vi "ShowData.vi"() -> ()   [LabVIEW 2022 SP3]
uses:
  <vilib>/sound2/lvsound2.llb/Sound Data Format.ctl
  <vilib>/sound2/lvsound2.llb/Sampling Mode.ctl
  <vilib>/sound2/lvsound2.llb/Sound Output Write (DBL Single).vi
panel:
  in  "Previous":bool
  in  "Next":bool
  out "Seek":bool
  out "TotSmpls":i64
  in  "PrevBtn":bool
  in  "SkipBtn":bool
  in  "FilePos":i32=8000
  in  "Skip":i32=220000 format="%#_4p"
  out "dt":dbl
  out "PlayBuffer":dbl[](array[numeric])
  out "Cnt":i32
  out "Chunks":i32
  in  "Export":path=path "D:/Temp"
  out "task ID":u32
  out "n":u16=1
  in  "ch":u16
  in  "ch_mask":u16=8000 format="%05b"
  in  "Reload":bool
  in  "SaveWav":bool
  in  "fs":u16=8000
  in  "Play":bool
  in  "Path":path
  out "min":u16
  out "max":u16
  out "Graph":u16[][](graph)
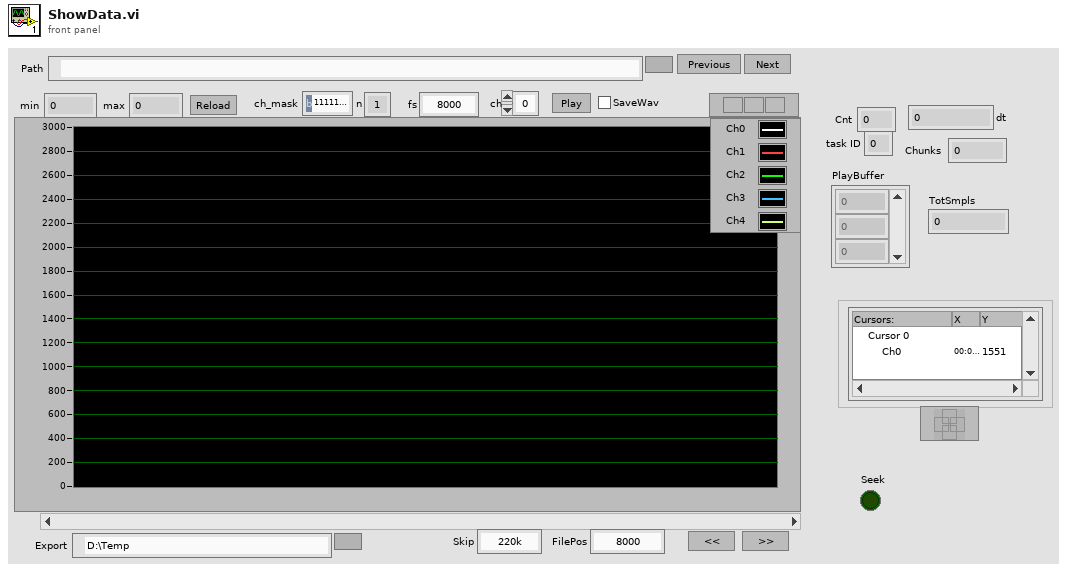
[diagram p1: front panel]
types:
  T1 = enum16{"big-endian, network order", "native, host order", "little-endian"}
  T2 = typedef "Sound Data Format.ctl" = cluster{"sample rate (S/s)":dbl, "number of channels":i32, "bits per sample":i32}
  T3 = typedef "Sampling Mode.ctl" = i32
  T4 = typedef "Sound Output Task ID.ctl" = u32
  T5 = typedef "LVPoint32TypeDef.ctl" = cluster{"Horizontal":i32, "Vertical":i32}
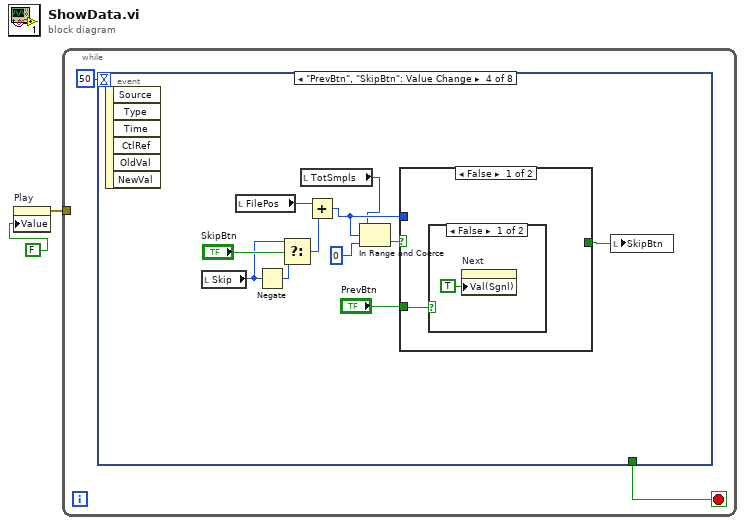
[diagram p0: block diagram]
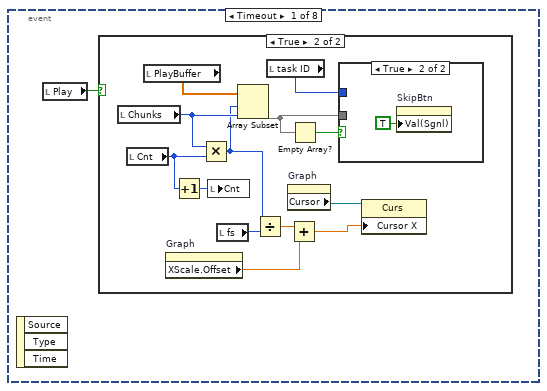
[diagram p2: hidden frame]
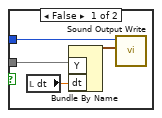
[diagram p4: hidden frame]
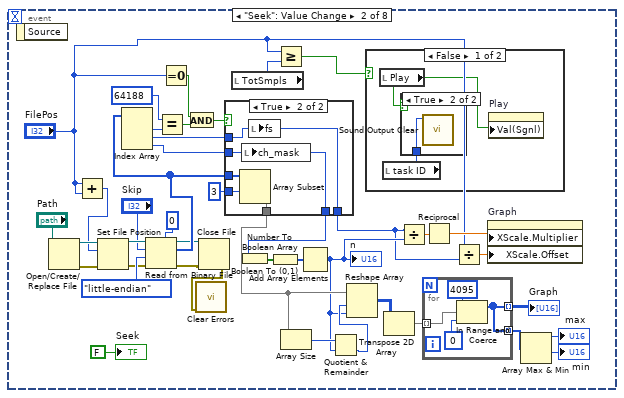
[diagram p5: hidden frame]
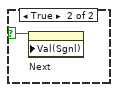
[diagram p7: hidden frame]
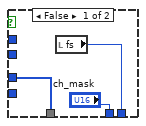
[diagram p8: hidden frame]
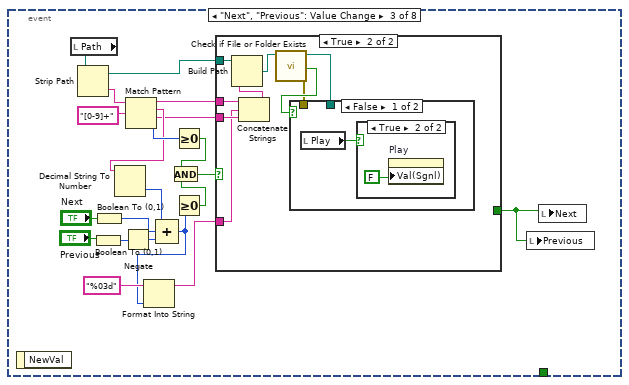
[diagram p9: hidden frame]
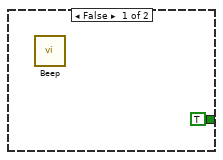
[diagram p10: hidden frame]
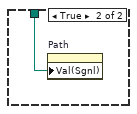
[diagram p12: hidden frame]
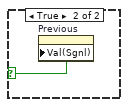
[diagram p13: hidden frame]
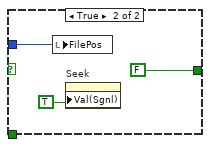
[diagram p14: hidden frame]
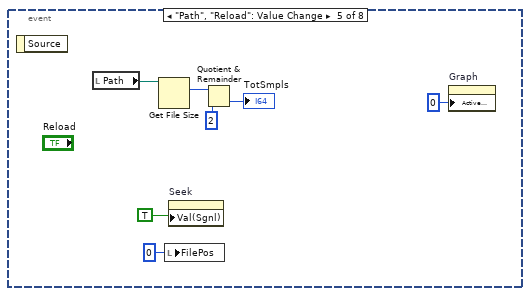
[diagram p15: hidden frame]
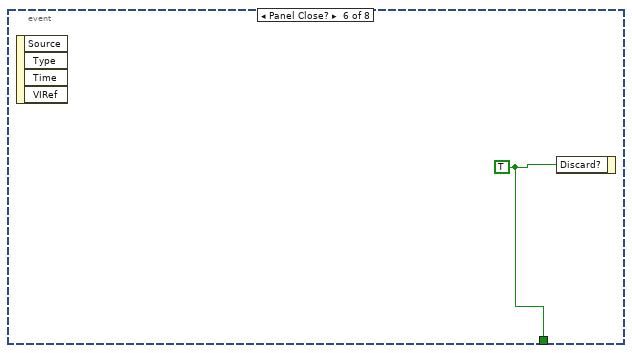
[diagram p16: hidden frame]
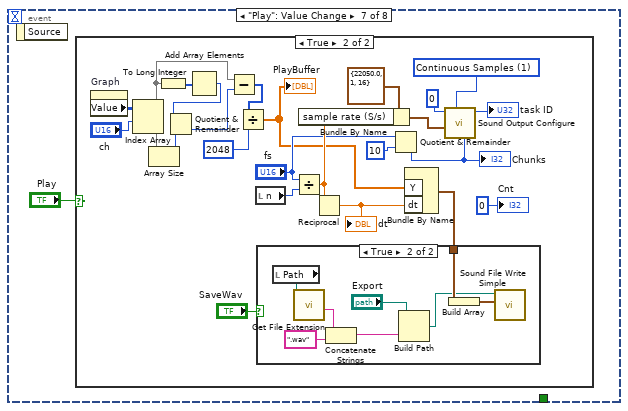
[diagram p17: hidden frame]
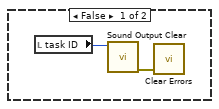
[diagram p18: hidden frame]
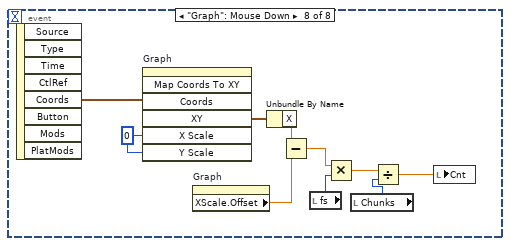
[diagram p20: hidden frame]
diagram:
  n1 = property on="Play" class="Bool (strict)"("Value"=FALSE) -> (error out=w2:errorcluster)  [unwired: 2 in, 1 out]
  n2 = while {
    tunnel: w2 -> [_]
    stop <- w4 stop-if-true
    n3 = event shown="[3] \"PrevBtn\", \"SkipBtn\": Value Change" {
      selector: _ -> [_ _ _ _ _ _ _ _]
      dyn-events: _ -> [_ _ _ _ _ _ _ _]
      timeout: 50 -> [_ _ _ _ _ _ _ _]
      tunnel: [_ _ _ _ _ w140 _ _] -> w4
      event Timeout {
        n4 = event-data() -> ()  [unwired: 1 in, 3 out]
        n5 = local read "Play"() -> (w5:bool)
        n6 = case shown="True" w5 {
          frame False {
          }
          frame True {
            n7 = local read "Chunks"() -> (w17:i32)
            n8 = local read "Cnt"() -> (w13:i32)
            n9 = local read "PlayBuffer"() -> (w18:dbl[])
            n10 = property on="Graph" class="WFGraph (strict)"() -> ("XScale.Offset"=w6:dbl)  [unwired: 2 in, 2 out]
            n11 = Increment(x=w13) -> (x+1=w12:i32)
            n12 = Multiply(x=w17, y=w13) -> (x*y=w10:i32)
            n13 = local write "Cnt"(w12) -> ()
            n14 = local read "fs"() -> (w11:u16)
            n15 = Array Subset(array=w18, index=w10, length=w17) -> (w15:dbl[])
            n16 = Divide(x=w10, y=w11) -> (x/y=w8:dbl)
            n17 = local read "task ID"() -> (w16:u32)
            n18 = property on="Graph" class="WFGraph (strict)"() -> ("Cursor"=w9:refnum<vi>)  [unwired: 2 in, 2 out]
            n19 = Add(x=w8, y=w6) -> (x+y=w7:dbl)
            n20 = Empty Array?(array=w15) -> (empty?=w14:bool)
            n21 = case shown="True" w14 {
              tunnel: w16 -> [w20 _]
              tunnel: w15 -> [w19 _]
              frame False {
                n22 = local read "dt"() -> (w22:dbl)
                n23 = Bundle By Name("Y"=w19, "dt"=w22) -> (w21:waveform(dbl))  [unwired: 1 in]
                n24 = call-poly <vilib>:"Sound Output Write.vi"("data"=w21, "task ID"=w20) -> ()  [unwired: 8 in, 2 out]
              }
              frame True {
                n25 = property on="SkipBtn" class="Bool (strict)"("Val(Sgnl)"=TRUE) -> ()  [unwired: 2 in, 2 out]
              }
            }
            n26 = property class="Curs"(reference=w9, "Cursor X"=w7) -> ()  [unwired: 1 in, 2 out]
          }
        }
      }
      event "Seek": Value Change {
        n27 = event-data() -> ()  [unwired: 1 in, 1 out]
        n28 = Open/Create/Replace File(file path (use dialog)="Path") -> (refnum out=w45:refnum<file>, error out=w42:errorcluster)  [unwired: 5 in, 1 out]
        n29 = Add(x="FilePos", y="FilePos") -> (x+y=w44:i32)
        n30 = Set File Position(offset (in bytes) (0)=w44, refnum=w45, error in=w42) -> (refnum out=w43:refnum<file>, error out=w27:errorcluster)  [unwired: 1 in]
        n31 = Read from Binary File(5:u16 0, 8:w27, 9:T1."little-endian" ("byte order (0:big-endian, network order)"), 10:"Skip", 11:w43) -> (0:w36:errorcluster, 2:w46:u16[], 3:w37:refnum<file>)  [unwired: 1 in, 1 out]
        n32 = Index Array(array=w46) -> (element #1=w59:u16, element #2=w57:u16, element #3=w56:u16)  [unwired: 3 in]
        n33 = Equal?(x=u16 64188, y=w59) -> (x = y?=w58:bool)
        n34 = Equal To 0?(x="FilePos") -> (x = 0?=w39:bool)
        n35 = And(x=w39, y=w58) -> (x .and. y?=w41:bool)
        n36 = Close File(refnum=w37, error in=w36) -> (error out=w28:errorcluster)  [unwired: 1 out]
        n37 = call <vilib>:"Clear Errors.vi"("error in (no error)"=w28) -> ()  [unwired: 5 in, 2 out]
        n38 = case shown="True" w41 {
          tunnel: w57 -> [_ w73]
          tunnel: w46 -> [w72 w77]
          tunnel: w56 -> [_ w74]
          tunnel: 3 ("index") -> [_ w76]
          tunnel: [w72 w75] -> w50
          tunnel: ["ch_mask" w74] -> w49
          tunnel: [w70 w73] -> w30
          frame False {
            n39 = local read "fs"() -> (w70:u16)
          }
          frame True {
            n40 = Array Subset(array=w77, index=w76) -> (w75:u16[])  [unwired: 1 in]
            n41 = local write "ch_mask"(w74) -> ()
            n42 = local write "fs"(w73) -> ()
          }
        }
        n43 = local read "TotSmpls"() -> (w35:i64)
        n44 = Number To Boolean Array(number=w49) -> (Boolean array=w54:bool[])
        n45 = Boolean To (0,1)(Boolean=w54) -> (0, 1=w53:i16[])
        n46 = Greater Or Equal?(x="FilePos", y=w35) -> (x >= y?=w25:bool)
        n47 = Array Size(array=w50) -> (size(s)=w52:i32)
        n48 = Add Array Elements(numeric array=w53) -> (sum=w34:i16)
        "n" <- w34
        n49 = Quotient & Remainder(x=w52, y=w34) -> (floor(x/y)=w48:i32)  [unwired: 1 out]
        n50 = Reshape Array(w50, w48, w34) -> (w51:u16[][])
        n51 = case shown="False" w25 {
          selector: w25 -> [_ w69]
          frame False {
            n52 = local read "Play"() -> (w66:bool)
            n53 = local read "task ID"() -> (w67:u32)
            n54 = case shown="True" w66 {
              tunnel: w67 -> [_ w68]
              frame False {
              }
              frame True {
                n55 = call <vilib>:"Sound Output Clear.vi"("task ID"=w68) -> ()  [unwired: 10 in, 1 out]
              }
            }
            n56 = property on="Play" class="Bool (strict)"("Val(Sgnl)"=w66) -> ()  [unwired: 2 in, 2 out]
          }
          frame True {
            n57 = property on="Next" class="Bool (strict)"("Val(Sgnl)"=w69) -> ()  [unwired: 2 in, 2 out]
          }
        }
        n58 = Transpose 2D Array(2D array=w51) -> (transposed array=w61:u16[][])
        n59 = Divide(x=w30, y=w34) -> (x/y=w33:dbl)
        n60 = for {
          tunnel: w61 -> [w79] mode=indexing
          tunnel: [w78] -> w63 mode=indexing
          tunnel: [w78] -> w62 mode=concatenating
          n61 = In Range and Coerce(upper limit=u16 4095 ("x"), x=w79, lower limit=u16 0 ("x")) -> (coerced(x)=w78:u16[])  [unwired: 1 out]
        }
        "Graph" <- w63
        n62 = Reciprocal(x=w33) -> (1/x=w32:dbl)
        n63 = Divide(x="FilePos", y=w30) -> (x/y=w31:dbl)
        n64 = property on="Graph" class="WFGraph (strict)"("XScale.Multiplier"=w32, "XScale.Offset"=w31) -> ()  [unwired: 2 in, 2 out]
        n65 = Array Max & Min(array=w62) -> (max value=→"max":u16, min value=→"min":u16)  [unwired: 2 out]
        "Seek" <- FALSE
      }
      event "Next", "Previous": Value Change {
        n66 = event-data() -> ()  [unwired: 1 in, 1 out]
        n67 = local read "Path"() -> (w97:path)
        n68 = Strip Path(path=w97) -> (stripped path=w91:path, name=w96:string)
        n69 = Boolean To (0,1)(Boolean="Previous") -> (0, 1=w100:i16)
        n70 = Boolean To (0,1)(Boolean="Next") -> (0, 1=w98:i16)
        n71 = Negate(x=w100) -> (-x=w99:i16)
        n72 = Match Pattern(string=w96, regular expression="[0-9]+") -> (before substring=w90:string, match substring=w93:string, after substring=w89:string, offset past match=w94:i32)  [unwired: 1 in]
        n73 = Decimal String To Number(string=w93) -> (number=w92:i32)  [unwired: 2 in, 1 out]
        n74 = Compound Arithmetic op=ADD(w92, w98, w99) -> (w83:i32)
        n75 = Format Into String(format string="%03d", w83) -> (resulting string=w87:string)  [unwired: 2 in, 1 out]
        n76 = Greater Or Equal To 0?(x=w94) -> (x >= 0?=w85:bool)
        n77 = Greater Or Equal To 0?(x=w83) -> (x >= 0?=w84:bool)
        n78 = And(x=w85, y=w84) -> (x .and. y?=w86:bool)
        n79 = case shown="True" w86 {
          tunnel: w91 -> [_ w112]
          tunnel: w90 -> [_ w110]
          tunnel: w89 -> [_ w109]
          tunnel: w87 -> [_ w108]
          tunnel: [TRUE _] -> w82
          frame False {
            n80 = call <vilib>:"Beep.vi"() -> ()  [unwired: 12 in]
          }
          frame True {
            n81 = Concatenate Strings(w110, w108, w109) -> (w111:string)
            n82 = Build Path(base path=w112, name or relative path=w111) -> (appended path=w107:path)
            n83 = call <vilib>:"Check if File or Folder Exists.vi"("path"=w107) -> ("error out"=w105:errorcluster, "file or folder exists?"=w106:bool, "dup path"=w104:path)  [unwired: 8 in]
            n84 = case shown="False" w106 {
              tunnel: w105 -> [_ _]
              tunnel: w104 -> [_ w115]
              frame False {
                n85 = local read "Play"() -> (w113:bool)
                n86 = case shown="True" w113 {
                  frame False {
                  }
                  frame True {
                    n87 = property on="Play" class="Bool (strict)"("Val(Sgnl)"=FALSE) -> ()  [unwired: 2 in, 2 out]
                  }
                }
              }
              frame True {
                n88 = property on="Path" class="Path"("Val(Sgnl)"=w115) -> ()  [unwired: 2 in, 2 out]
              }
            }
          }
        }
        n89 = local write "Previous"(w82) -> ()
        n90 = local write "Next"(w82) -> ()
      }
      event "PrevBtn", "SkipBtn": Value Change {
        n91 = event-data() -> ()  [unwired: 1 in, 6 out]
        n92 = local read "Skip"() -> (w123:i32)
        n93 = local read "FilePos"() -> (w126:i32)
        n94 = Negate(x=w123) -> (-x=w125:i32)
        n95 = Select(t=w123, s="SkipBtn", f=w125) -> (s? t:f=w122:i32)
        n96 = local read "TotSmpls"() -> (w117:i64)
        n97 = Add(x=w126, y=w122) -> (x+y=w119:i32)
        n98 = In Range and Coerce(upper limit=w117, x=w119, lower limit=0) -> (In Range?=w121:bool)  [unwired: 1 out]
        n99 = case shown="False" w121 {
          tunnel: w119 -> [_ w131]
          tunnel: [_ FALSE] -> w120
          tunnel: "PrevBtn" -> [w127 _]
          frame False {
            n100 = case shown="False" w127 {
              selector: w127 -> [_ w129]
              frame False {
                n101 = property on="Next" class="Bool (strict)"("Val(Sgnl)"=TRUE) -> ()  [unwired: 2 in, 2 out]
              }
              frame True {
                n102 = property on="Previous" class="Bool (strict)"("Val(Sgnl)"=w129) -> ()  [unwired: 2 in, 2 out]
              }
            }
          }
          frame True {
            n103 = local write "FilePos"(w131) -> ()
            n104 = property on="Seek" class="Bool (strict)"("Val(Sgnl)"=TRUE) -> ()  [unwired: 2 in, 2 out]
          }
        }
        n105 = local write "SkipBtn"(w120) -> ()
      }
      event "Path", "Reload": Value Change {
        n106 = event-data() -> ()  [unwired: 1 in, 1 out]
        n107 = local read "Path"() -> (w137:path)
        n108 = Get File Size(file=w137) -> (size (in bytes)=w135:i64)  [unwired: 1 in, 2 out]
        n109 = local write "FilePos"(0 ("FilePos")) -> ()
        n110 = property on="Seek" class="Bool (strict)"("Val(Sgnl)"=TRUE) -> ()  [unwired: 2 in, 2 out]
        n111 = Quotient & Remainder(x=w135, y=i64 2) -> (floor(x/y)=→"TotSmpls":i64)  [unwired: 1 out]
        n112 = property on="Graph" class="WFGraph (strict)"("Active Cursor"=u32 0) -> ()  [unwired: 2 in, 2 out]
      }
      event Panel Close? {
        w140 = TRUE
        n113 = event-data() -> ()  [unwired: 1 in, 4 out]
        n114 = event-data("Discard?"=w140) -> ()  [unwired: 1 in, 1 out]
      }
      event "Play": Value Change {
        n115 = event-data() -> ()  [unwired: 1 in, 1 out]
        n116 = case shown="True" "Play" {
          frame False {
            n117 = local read "task ID"() -> (w143:u32)
            n118 = call <vilib>:"Sound Output Clear.vi"("task ID"=w143) -> ("error out"=w142:errorcluster)  [unwired: 10 in]
            n119 = call <vilib>:"Clear Errors.vi"("error in (no error)"=w142) -> ()  [unwired: 5 in, 2 out]
          }
          frame True {
            w157 = T3 1 items=["Finite Samples", "Continuous Samples"] ("sample mode")
            n120 = property on="Graph" class="WFGraph (strict)"() -> ("Value"=w165:u16[][])  [unwired: 2 in, 2 out]
            n121 = Index Array(array=w165, index (row)="ch") -> (element=w148:u16[])  [unwired: 1 in]
            n122 = Array Size(array=w148) -> (size(s)=w156:i32)
            n123 = To Long Integer(number=w148) -> (32bit integer=w150:i32[])
            n124 = Add Array Elements(numeric array=w150) -> (sum=w149:i32)
            n125 = Quotient & Remainder(x=w149, y=w156) -> (floor(x/y)=w147:i32)  [unwired: 1 out]
            n126 = Subtract(x=w148, y=w147) -> (x-y=w146:i32[])
            n127 = Divide(x=w146, y=2048) -> (x/y=w144:dbl[])
            "PlayBuffer" <- w144
            n128 = local read "n"() -> (w163:u16)
            n129 = Divide(x="fs", y=w163) -> (x/y=w160:dbl)
            n130 = Bundle By Name(cluster=T2 {"sample rate (S/s)"=22050.0, "number of channels"=1, "bits per sample"=16} ("sound format"), "sample rate (S/s)"=w160) -> (w161:T2)
            n131 = Reciprocal(x=w160) -> (1/x=w167:dbl)
            "dt" <- w167
            n132 = Quotient & Remainder(x="fs", y=u16 10) -> (floor(x/y)=w153:u16)  [unwired: 1 out]
            "Chunks" <- w153
            n133 = Bundle By Name("Y"=w144, "dt"=w167) -> (w159:waveform(dbl))  [unwired: 1 in]
            n134 = case shown="True" "SaveWav" {
              tunnel: w159 -> [_ w171]
              frame False {
              }
              frame True {
                n135 = local read "Path"() -> (w175:path)
                n136 = call <vilib>:"Get File Extension.vi"("file"=w175) -> ("filename without extension"=w173:string)  [unwired: 6 in, 4 out]
                n137 = Concatenate Strings(w173, ".wav" ("string")) -> (w174:string)
                n138 = Build Path(base path="Export", name or relative path=w174) -> (appended path=w169:path)
                n139 = Build Array(w171) -> (w170:waveform(dbl)[])
                n140 = call <vilib>:"Sound File Write Simple.vi"("data"=w170, "path"=w169) -> ()  [unwired: 8 in, 2 out]
              }
            }
            n141 = call <vilib>:"Sound Output Configure.vi"("number of samples/ch"=w153, "sample mode"=w157, "sound format"=w161, "device ID"=u32 0) -> ("task ID"=→"task ID":T4)  [unwired: 6 in, 1 out]
            "Cnt" <- u16 0 ("Cnt")
          }
        }
      }
      event "Graph": Mouse Down {
        w184 = 0 ("X Scale")
        n142 = event-data() -> ("Coords"=w185:T5)  [unwired: 1 in, 7 out]
        n143 = invoke on="Graph" class="WFGraph (strict)" method="Map Coords To XY"("Coords"=w185, "X Scale"=w184, "Y Scale"=w184) -> ("XY"=w183:cluster{"X":dbl, "Y":dbl})  [unwired: 4 in, 6 out]
        n144 = property on="Graph" class="WFGraph (strict)"() -> ("XScale.Offset"=w181:dbl)  [unwired: 2 in, 2 out]
        n145 = Unbundle By Name(w183) -> ("X"=w182:dbl)
        n146 = Subtract(x=w182, y=w181) -> (x-y=w180:dbl)
        n147 = local read "fs"() -> (w179:u16)
        n148 = Multiply(x=w180, y=w179) -> (x*y=w178:dbl)
        n149 = local read "Chunks"() -> (w177:i32)
        n150 = Divide(x=w178, y=w177) -> (x/y=w176:dbl)
        n151 = local write "Cnt"(w176) -> ()
      }
    }
  }
